vi "Func_CheckIfTypeExists.vi"(8 "error in (no error)":errorcluster, 11 "data type name":string) -> (0 "error out":errorcluster, 3 "Exists":bool)   [LabVIEW 2010, in "TemplateGenerator.lvlib"]
uses:
  TemplateGenerator.lvlib
  Type Defs/Data Types.ctl
  Current Value Table.lvlib
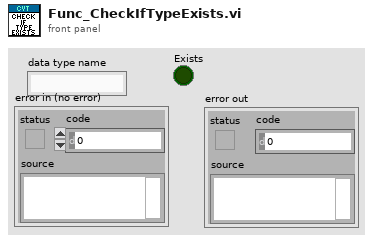
[diagram p1: front panel]
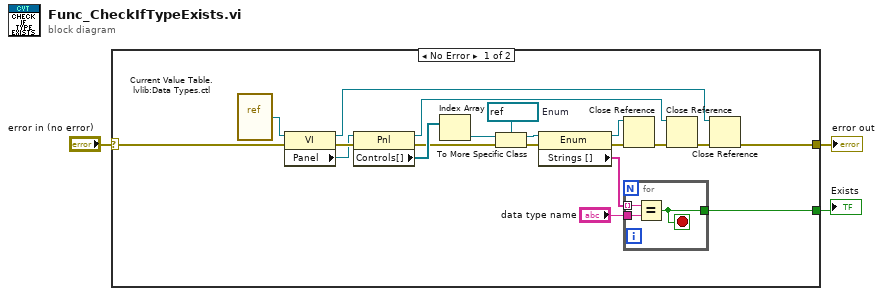
[diagram p0: block diagram]
diagram:
  n1 = case shown="No Error" "error in (no error)" {
    selector: "error in (no error)" -> [w5 w27]
    tunnel: [w6 w27] -> w3
    tunnel: [w4 _] -> w1
    frame No Error {
      w15 = refnum<vi> refnum  # Enum
      n2 = vi-ref "Current Value Table.lvlib:Data Types.ctl"() -> (w7:refnum<vi>)
      n3 = property class="VI"(reference=w7, error in=w5) -> (reference out=w13:refnum<vi>, error out=w14:errorcluster, "Panel"=w8:refnum<vi>)
      n4 = property class="Pnl"(reference=w8, error in=w14) -> (reference out=w11:refnum<vi>, error out=w9:errorcluster, "Controls[]"=w20:refnum<vi>[])
      n5 = Index Array(array=w20) -> (element=w21:refnum<vi>)  [unwired: 1 in]
      n6 = To More Specific Class(target class=w15, reference=w21, error in=w9) -> (specific class reference=w16:refnum<vi>, error out=w19:errorcluster)
      n7 = property class="Enum"(reference=w16, error in=w19) -> (reference out=w18:refnum<vi>, error out=w17:errorcluster, "Strings []"=w22:string[])
      n8 = Close Reference(reference=w18, error in (no error)=w17) -> (error out=w10:errorcluster)
      n9 = for {
        tunnel: w22 -> [w26] mode=indexing
        tunnel: "data type name" -> [w25]
        tunnel: [w24] -> w4
        stop <- w24 stop-if-true
        n10 = Equal?(x=w26, y=w25) -> (x = y?=w24:bool)
      }
      n11 = Close Reference(reference=w11, error in (no error)=w10) -> (error out=w12:errorcluster)
      n12 = Close Reference(reference=w13, error in (no error)=w12) -> (error out=w6:errorcluster)
    }
    frame Error {
    }
  }
  "error out" <- w3
  "Exists" <- w1
